vi "GetParam.vi"(8 "error in (no error)":errorcluster caption="entrée d'erreur (pas d'erreur)", 11 "Hinge_Loss.lvclass":refnum<class "Hinge_Loss.lvclass">) -> (0 "error out":errorcluster caption="sortie d'erreur", 2 "hinge_loss":cluster{"labels":i32[], "sample_weight":dbl[]}, 3 "Hinge_Loss.lvclass":refnum<class "Hinge_Loss.lvclass">)   [LabVIEW 2020, in "Hinge_Loss.lvclass"]
doc: "Get Parameters"
uses:
  Hinge_Loss.lvclass
  Hinge_Loss.lvclass/Hinge_Loss.ctl
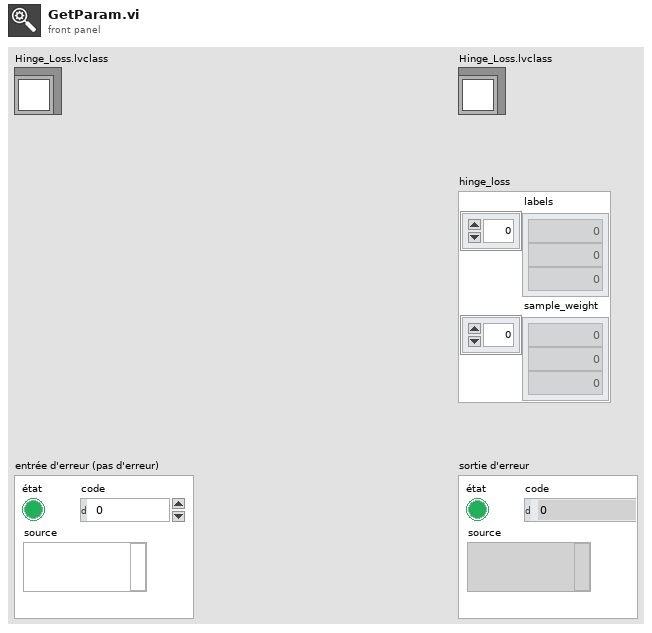
[diagram p1: front panel]
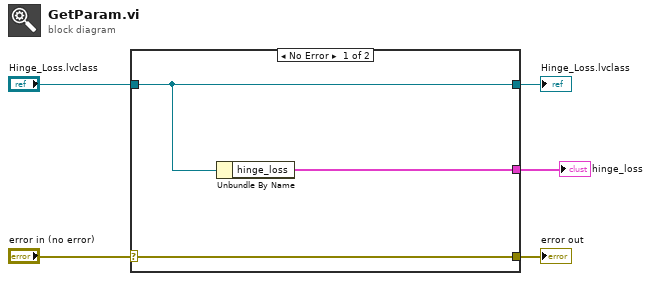
[diagram p0: block diagram]
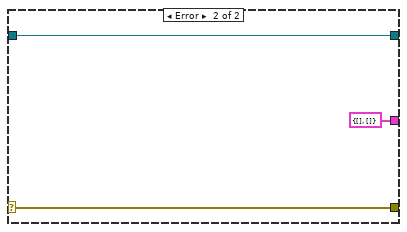
[diagram p2: hidden frame]
diagram:
  n1 = case shown="No Error" "error in (no error)" {
    selector: "error in (no error)" -> [w8 w10]
    tunnel: [w8 w10] -> w4
    tunnel: [w7 w11] -> w2
    tunnel: "Hinge_Loss.lvclass" -> [w7 w11]
    tunnel: [w6 cluster{"labels":i32[], "sample_weight":dbl[]} {"labels"=[], "sample_weight"=[]} ("hinge_loss")] -> w1
    frame No Error {
      n2 = Unbundle By Name(w7) -> ("hinge_loss"=w6:cluster{"labels":i32[], "sample_weight":dbl[]})
    }
    frame Error {
    }
  }
  "error out" <- w4
  "Hinge_Loss.lvclass" <- w2
  "hinge_loss" <- w1
